vi "DPO4034 Channel Enable.vi"(8 "error in (no error)":errorcluster, 10 "Channel (0: Channel 1)":u16(ring) items=["Channel 1", "Channel 2", "Channel 3", "Channel 4", "Math", "Reference 1", "Reference 2", "Reference 3", "Reference 4"], 11 "VISA resource name":refnum<visa-resource-name>) -> (0 "error out":errorcluster, 2 "Enabled":bool, 3 "VISA resource name out":refnum<visa-resource-name>)   [LabVIEW 2012]
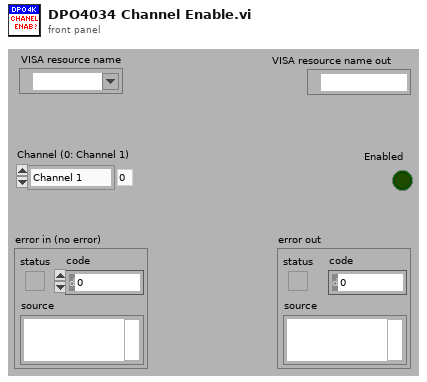
[diagram p1: front panel]
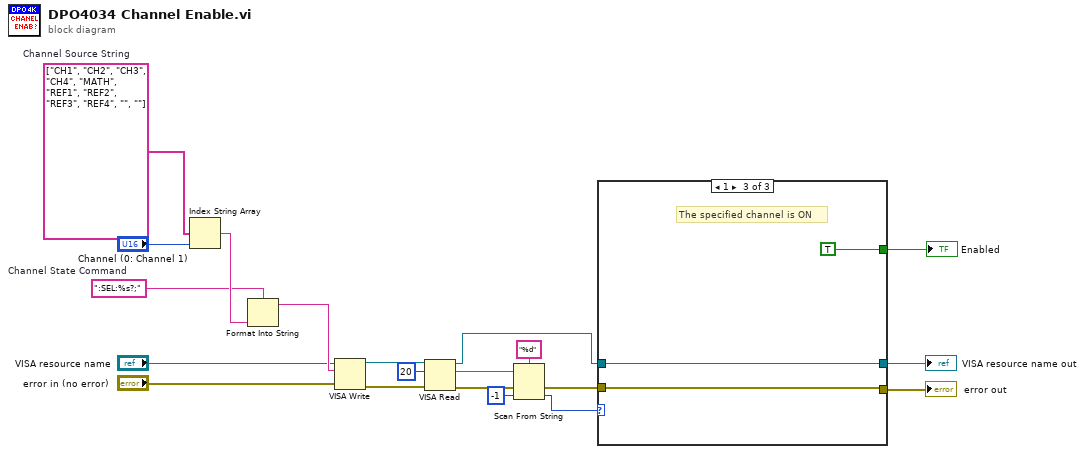
[diagram p0: block diagram]
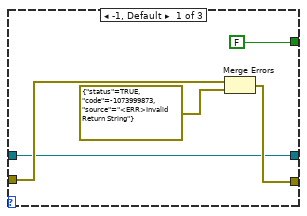
[diagram p2: hidden frame]
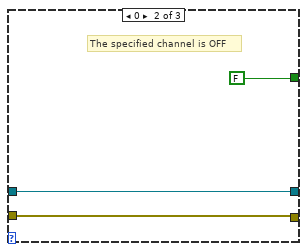
[diagram p3: hidden frame]
diagram:
  w4 = ":SEL:%s?;"  # Channel State Command
  w3 = string[] ["CH1", "CH2", "CH3", "CH4", "MATH", "REF1", "REF2", "REF3", "REF4", "", ""]  # Channel Source String
  n1 = Index String Array(1:"Channel (0: Channel 1)", 2:w3) -> (0:w5:string)  [unwired: 1 in]
  n2 = Format Into String(format string=w4, w5) -> (resulting string=w8:string)  [unwired: 2 in, 1 out]
  n3 = VISA Write(VISA resource name="VISA resource name", write buffer=w8, error in (no error)="error in (no error)") -> (VISA resource name out=w9:refnum<visa-resource-name>, error out=w10:errorcluster)  [unwired: 1 out]
  n4 = VISA Read(VISA resource name=w9, byte count=u32 20, error in (no error)=w10) -> (VISA resource name out=w18:refnum<visa-resource-name>, read buffer=w14:string, error out=w15:errorcluster)  [unwired: 1 out]
  n5 = Scan From String(format string="%d", input string=w14, error in=w15, default 1=-1 ("default value 1")) -> (error out=w17:errorcluster, output 1=w20:i32)  [unwired: 1 in, 2 out]
  n6 = case shown="1" w20 {
    tunnel: w18 -> [w22 w28 w31]
    tunnel: w17 -> [w24 w27 w29]
    tunnel: [w23 w27 w29] -> w13
    tunnel: [w22 w28 w31] -> w12
    tunnel: [FALSE FALSE TRUE] -> w1
    frame -1, Default {
      n7 = Merge Errors(w24, errorcluster {"status"=TRUE, "code"=-1073999873, "source"="<ERR>Invalid Return String"} ("error out")) -> (w23:errorcluster)
    }
    frame 0 {
      # "The specified channel is OFF"
    }
    frame 1 {
      # "The specified channel is ON"
    }
  }
  "error out" <- w13
  "VISA resource name out" <- w12
  "Enabled" <- w1
